vi "Create User Que.vi"(7 "最大キューサイズ（-1, 無制限）":i32=-1, 8 "error in":errorcluster) -> (0 "error out":errorcluster, 3 "queVariant":refnum<queue>)   [LabVIEW 2014]
uses:
  QueData.ctl
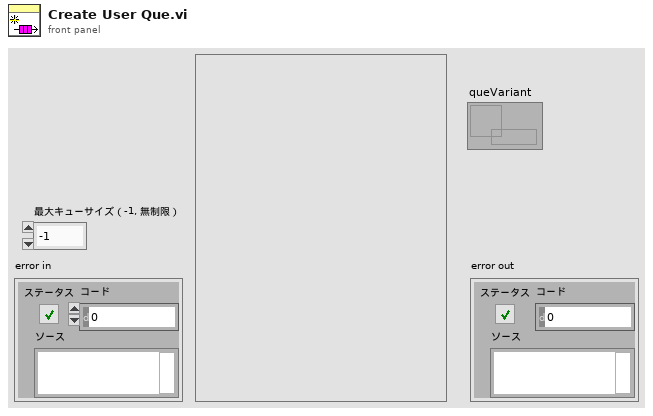
[diagram p1: front panel]
types:
  T1 = typedef "QueData.ctl" = cluster{"コマンド":string, "バリアント":variant}
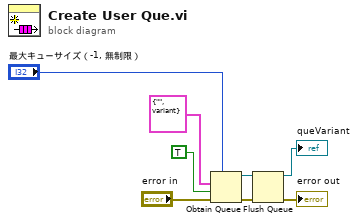
[diagram p0: block diagram]
diagram:
  n1 = Obtain Queue(max queue size (-1, unlimited)="最大キューサイズ（-1, 無制限）", element data type=T1 {"コマンド"="", "バリアント"=variant}, create if not found? (T)=TRUE, error in (no error)="error in") -> (queue out=w5:refnum<queue>, error out=w6:errorcluster)  [unwired: 1 in, 1 out]
  n2 = Flush Queue(queue=w5, error in (no error)=w6) -> (queue out=→"queVariant":refnum<queue>, error out=→"error out":errorcluster)  [unwired: 1 out]
